vi "Set Shutter.vi"(8 "error in (no error)":errorcluster, 11 "CCDCamera in":refnum<class "Real Camera.lvclass">) -> (0 "error out":errorcluster, 3 "CCDCamera out":refnum<class "Real Camera.lvclass">)   [LabVIEW 2018, in "Real Camera.lvclass"]
doc: "Set the shutter configuration\n\nWith this function, the shutter mode as well as the shutter opening and closing times can be set."
uses:
  Real Camera.lvclass
  C:/Users/Denis/Desktop/S4ACS/S4ACS/Simulated_CCD_Camera/Simulated Camera.lvclass
  Simulated_CCD_Camera/Simulated Camera.lvclass
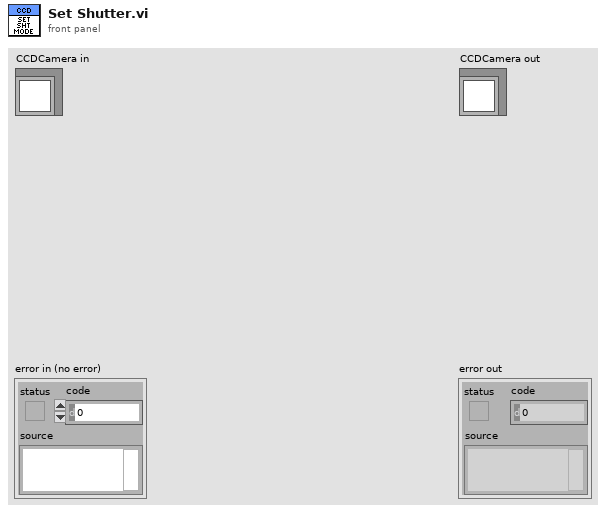
[diagram p1: front panel]
types:
  T1 = cluster{"PREAMP":u16, "READOUT_RATE":u16, "EM_GAIN":u16, "VERTICAL_SHIFT_SPEED":u16, "READ_MODE":u16, "FRAME_TRANSFER":bool, "VERTICAL_CLOCK_VOLTAGE":u16, "ACQUISITION_MODE":u16, "AD_CHANNEL":u16, "EM_MODE":u16, "SHUTTER_TTL":u16, "SHUTTER_OPENING_TIME":u16, "SHUTTER_CLOSING_TIME":u16, "SHUTTER_MODE":u16, "TRIGGER_MODE":u16, "VBIN":u16, "INITIAL_LINE":u16, "INITIAL_COLUMN":u16, "FINAL_LINE":u16, "FINAL_COLUMN":u16, "HBIN":u16}
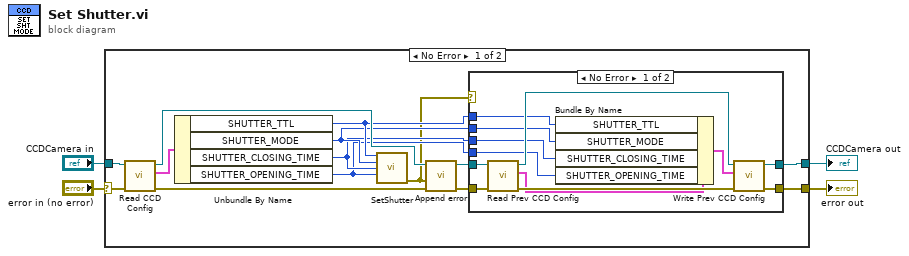
[diagram p0: block diagram]
diagram:
  n1 = case shown="No Error" "error in (no error)" {
    selector: "error in (no error)" -> [w18 w34]
    tunnel: [w10 w34] -> w4
    tunnel: [w11 w33] -> w3
    tunnel: "CCDCamera in" -> [w16 w33]
    frame No Error {
      n2 = call "Read CCD Config.vi"("error in (no error)"=w18, "CCDCamera in"=w16) -> ("error out"=w14:errorcluster, "CCD Config"=w17:T1, "CCDCamera out"=w15:refnum<class "Real Camera.lvclass">)  [unwired: 7 in]
      n3 = Unbundle By Name(w17) -> ("SHUTTER_TTL"=w9:u16, "SHUTTER_MODE"=w8:u16, "SHUTTER_CLOSING_TIME"=w7:u16, "SHUTTER_OPENING_TIME"=w6:u16)
      n4 = call <userlib>:"SetShutter.vi"("type"=w9, "mode"=w8, "closingtime"=w7, "openingtime"=w6) -> ("error out"=w5:errorcluster)  [unwired: 10 in, 1 out]
      n5 = call "Append error.vi"("error in (no error)"=w14, "error"=w5, "Simulated_CCD_Camera in"=w15) -> ("error out"=w12:errorcluster, "Simulated_CCD_Camera out"=w13:refnum<class "Real Camera.lvclass">)  [unwired: 7 in]
      n6 = case shown="No Error" w5 {
        tunnel: [w29 w32] -> w11
        tunnel: [w27 w31] -> w10
        tunnel: w13 -> [w24 w32]
        tunnel: w12 -> [w23 w31]
        tunnel: w9 -> [w22 _]
        tunnel: w8 -> [w21 _]
        tunnel: w7 -> [w20 _]
        tunnel: w6 -> [w19 _]
        frame No Error {
          n7 = call-dynamic "Read Prev CCD Config.vi"("error in (no error)"=w23, "Simulated_CCD_Camera in"=w24) -> ("error out"=w28:errorcluster, "Prev CCD Config"=w26:T1, "Simulated_CCD_Camera out"=w30:refnum<class "Real Camera.lvclass">)  [unwired: 7 in]
          n8 = Bundle By Name(cluster=w26, "SHUTTER_TTL"=w22, "SHUTTER_MODE"=w21, "SHUTTER_CLOSING_TIME"=w20, "SHUTTER_OPENING_TIME"=w19) -> (w25:T1)
          n9 = call-dynamic "Write Prev CCD Config.vi"("error in (no error)"=w28, "Prev CCD Config"=w25, "Simulated_CCD_Camera in"=w30) -> ("error out"=w27:errorcluster, "Simulated_CCD_Camera out"=w29:refnum<class "Real Camera.lvclass">)  [unwired: 7 in]
        }
        frame Error {
        }
      }
    }
    frame Error {
    }
  }
  "error out" <- w4
  "CCDCamera out" <- w3
